vi "EditorUndoRedoNewItem.vi"(8 "error in (no error)":errorcluster, 9 "Data in":variant, 10 "Message":string, 11 "UndoRedoCluster":T1) -> (0 "error out":errorcluster)   [LabVIEW 2020]
uses:
  TypeDef/EditorUndoRedoCluster.ctl
  MessageQueue/QueueRef.ctl
  MessageQueue/MessageQueue.lvlib
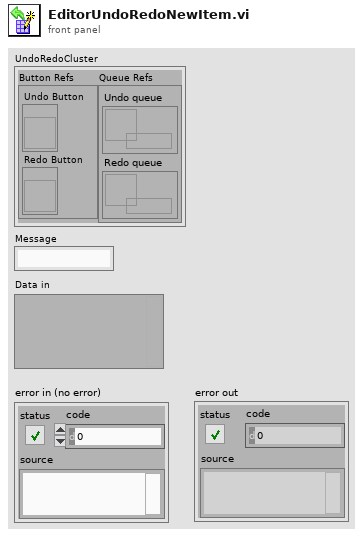
[diagram p1: front panel]
types:
  T1 = typedef "EditorUndoRedoCluster.ctl" = cluster{"Button Refs":cluster{"Undo Button":refnum<vi>, "Redo Button":refnum<vi>}, "Queue Refs":cluster{"Undo queue":T2, "Redo queue":T2}}
  T2 = typedef "MessageQueue.lvlib/QueueRef.ctl" = refnum<queue>
  T3 = enum8{"Enabled", "Disabled", "Disabled and Grayed Out"}
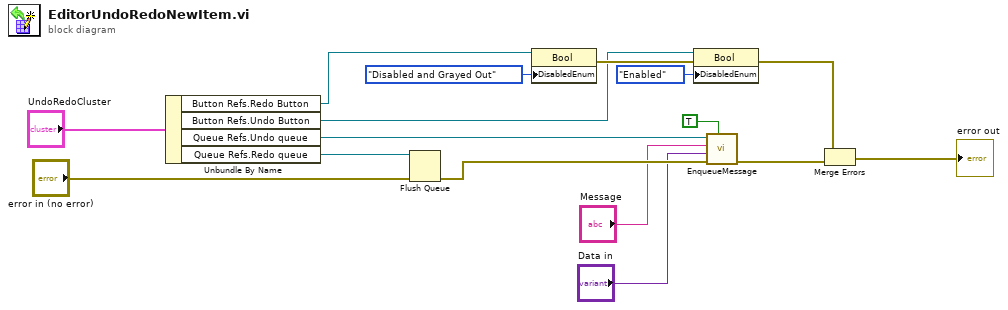
[diagram p0: block diagram]
diagram:
  n1 = Unbundle By Name("UndoRedoCluster") -> ("Button Refs.Redo Button"=w8:refnum<vi>, "Button Refs.Undo Button"=w9:refnum<vi>, "Queue Refs.Undo queue"=w4:T2, "Queue Refs.Redo queue"=w6:T2)
  n2 = Flush Queue(queue=w6, error in (no error)="error in (no error)") -> (error out=w7:errorcluster)  [unwired: 2 out]
  n3 = property class="Bool"(reference=w8, "DisabledEnum"=T3."Disabled and Grayed Out" ("Disabled")) -> (error out=w10:errorcluster)  [unwired: 1 in, 1 out]
  n4 = property class="Bool"(reference=w9, error in=w10, "DisabledEnum"=T3."Enabled" ("Disabled")) -> (error out=w13:errorcluster)  [unwired: 1 out]
  n5 = call "EnqueueMessage.vi"("Priority? (F)"=TRUE, "error in (no error)"=w7, "Data"="Data in", "Message"="Message", "queue in"=w4) -> ("error out"=w16:errorcluster)  [unwired: 5 in, 1 out]
  n6 = Merge Errors(w13, w16) -> (→"error out":errorcluster)
